vi "VITester_Global_Init.vi"(11 "Object":T1) -> ()   [LabVIEW 2013]
uses:
  <resource>/Framework/Providers/vitester-src/Support/VITester Project Item Ref.ctl
  <resource>/Framework/Providers/API/mxLvMenuItem.ctl
  <resource>/Framework/Providers/API/mxLvOverlayAlias.ctl
panel:
  out "error out":errorcluster
  in  "error in":errorcluster
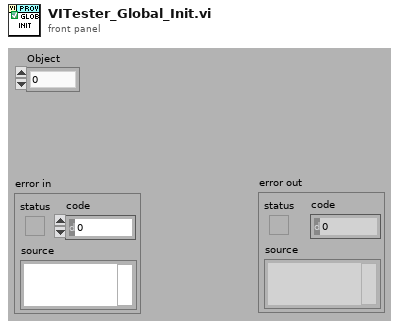
[diagram p1: front panel]
types:
  T1 = typedef "VITester Project Item Ref.ctl" = u64
  T2 = typedef "mxLvMenuItem.ctl" = cluster{"Menu Name":string, "Description":string, "Icon File Name":path, "Menu Tag":string, "Enabled":bool, "Checked":bool, "Separator":bool, "Batchable":bool, "Weight":i32, "Batch Mode (Ignored if Not Batchable)":enum32{"Show If All Items Support Command", "Show If Any Items Support Command"}, "Menu Location":enum32{"<None>", "Project", "Project / Build Specifications", "Tools", "Tools / Source Control", "Tools / Real-Time Module", "Help"}, "Exclude From Getting Started Window Menu":bool}
  T3 = typedef "ItemRef.ctl" = u64
  T4 = typedef "mxLvOverlayAlias.ctl" = cluster{"Overlay Alias":string, "Icon File Name":path}
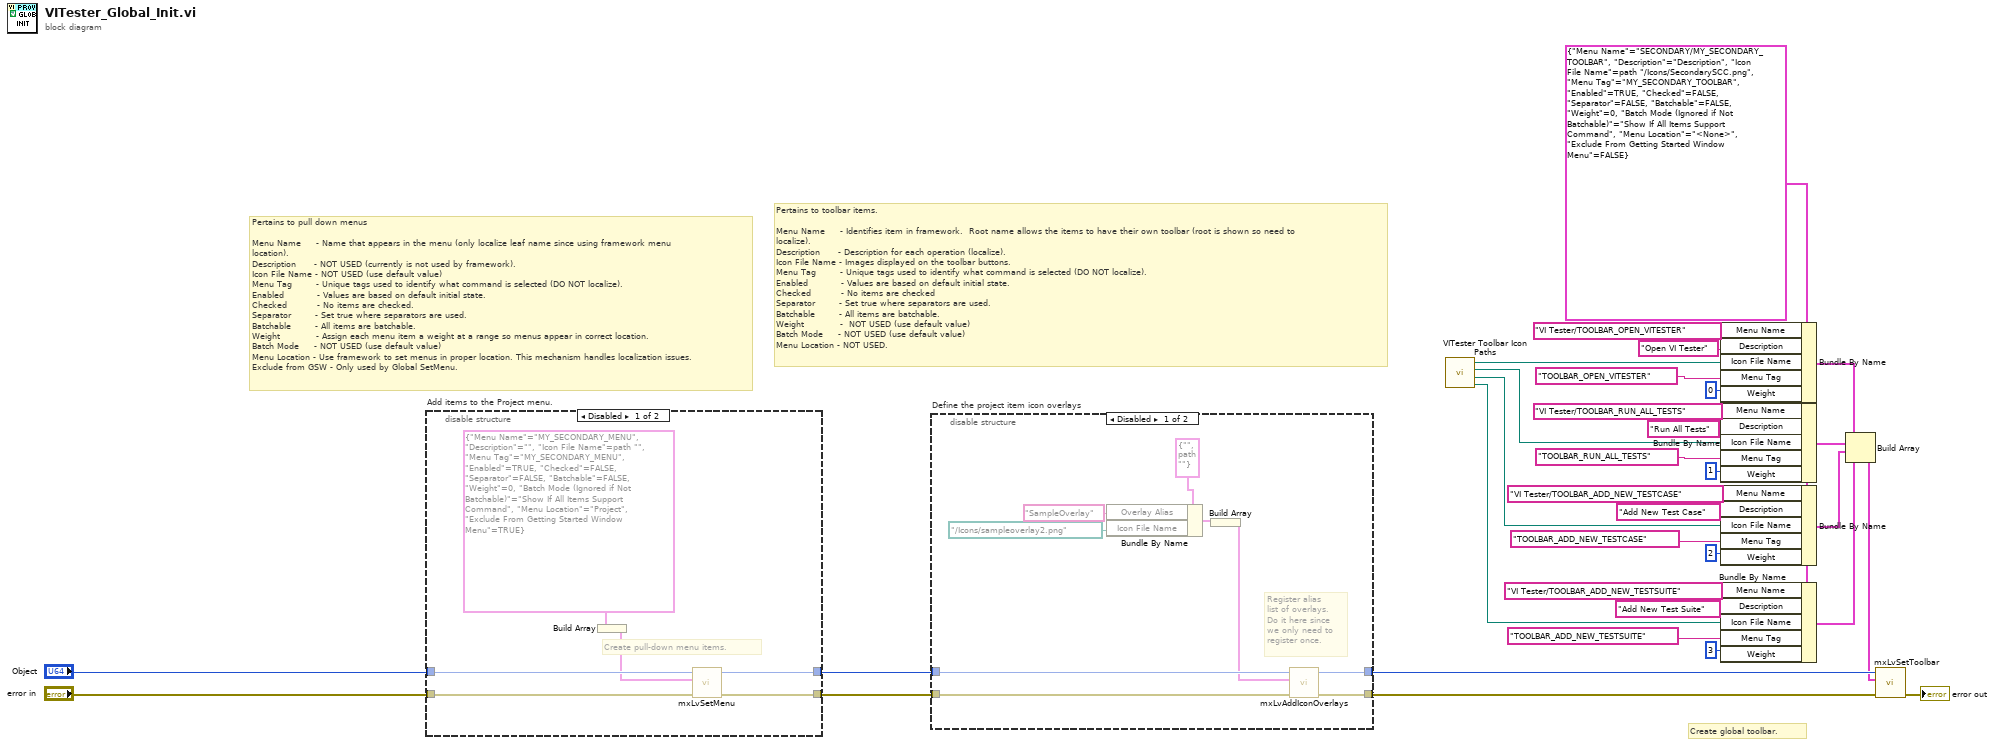
[diagram p0: block diagram]
diagram:
  w2 = T2 {"Menu Name"="SECONDARY/MY_SECONDARY_TOOLBAR", "Description"="Description", "Icon File Name"=path "../Icons/SecondarySCC.png", "Menu Tag"="MY_SECONDARY_TOOLBAR", "Enabled"=TRUE, "Checked"=FALSE, "Separator"=FALSE, "Batchable"=FALSE, "Weight"=0, "Batch Mode (Ignored if Not Batchable)"=enum."Show If All Items Support Command", "Menu Location"=enum."<None>", "Exclude From Getting Started Window Menu"=FALSE} ("Menu Item")
  # "Pertains to toolbar items.\n\nMenu Name     - Identifies item in framework.  Root name allows the items to have their own toolbar (root is shown so need to localize).\nDescription      - Description for each operation (localize).\nIcon File Name - Images displayed on the toolbar buttons.\nMenu Tag        - Unique tags used to identify what command is selected (DO NOT localize).\nEnabled           - Values are based on default initial state.\nChecked          - No items are checked\nSeparator        - Set true where separators are used.\nBatchable        - All items are batchable.\nWeight            -  NOT USED (use default value)\nBatch Mode     - NOT USED (use default value)\nMenu Location - NOT USED."
  # "Pertains to pull down menus\n\nMenu Name     - Name that appears in the menu (only localize leaf name since using framework menu location).\nDescription      - NOT USED (currently is not used by framework).\nIcon File Name - NOT USED (use default value)\nMenu Tag        - Unique tags used to identify what command is selected (DO NOT localize).\nEnabled           - Values are based on default initial state.\nChecked          - No items are checked.\nSeparator        - Set true where separators are used.\nBatchable        - All items are batchable.\nWeight            - Assign each menu item a weight at a range so menus appear in correct location.\nBatch Mode     - NOT USED (use default value)\nMenu Location - Use framework to set menus in proper location. This mechanism handles localization issues.\nExclude from GSW - Only used by Global SetMenu."
  # "Create global toolbar."
  n1 = disable-structure "Add items to the Project menu." shown="Disabled" {
    disable-tunnel: "error in" -> [w39 w40]
    disable-tunnel: [w38 w40] -> w32
    disable-tunnel: [w37 w41] -> w31
    disable-tunnel: "Object" -> [w36 w41]
    frame Disabled {
      # "Create pull-down menu items."
      n2 = Build Array(T2 {"Menu Name"="MY_SECONDARY_MENU", "Description"="", "Icon File Name"=path "", "Menu Tag"="MY_SECONDARY_MENU", "Enabled"=TRUE, "Checked"=FALSE, "Separator"=FALSE, "Batchable"=FALSE, "Weight"=0, "Batch Mode (Ignored if Not Batchable)"=enum."Show If All Items Support Command", "Menu Location"=enum."Project", "Exclude From Getting Started Window Menu"=TRUE} ("Menu Item")) -> (w34:T2[])
      n3 = call <resource>:"mxLvSetMenu.vi"("error in"=w39, "Menu Items"=w34, "Item"=w36) -> ("error out"=w38:errorcluster, "Item"=w37:T3)  [unwired: 7 in]
    }
    frame Enabled {
    }
  }
  n4 = disable-structure "Define the project item icon overlays" shown="Disabled" {
    disable-tunnel: w32 -> [w50 w51]
    disable-tunnel: w31 -> [w49 w52]
    disable-tunnel: [w48 w52] -> w30
    disable-tunnel: [w47 w51] -> w29
    frame Disabled {
      # "Register alias list of overlays.  Do it here since we only need to register once."
      n5 = Bundle By Name(cluster=T4 {"Overlay Alias"="", "Icon File Name"=path ""} ("Icon Overlay Alias"), "Overlay Alias"="SampleOverlay", "Icon File Name"=path "../Icons/sampleoverlay2.png") -> (w45:T4)
      n6 = Build Array(w45) -> (w44:T4[])
      n7 = call <resource>:"mxLvAddIconOverlays.vi"("error in"=w50, "Overlay Aliases"=w44, "Item"=w49) -> ("error out"=w47:errorcluster, "Item"=w48:T3)  [unwired: 7 in]
    }
    frame Enabled {
    }
  }
  n8 = call <resource>:"VITester Toolbar Icon Paths.vi"() -> ("Add New TestSuite toolbar icon"=w5:path, "Add New TestCase toolbar icon"=w17:path, "Run All Tests toolbar icon"=w12:path, "Open VI Tester toolbar icon"=w22:path)  [unwired: 8 in]
  n9 = Bundle By Name(cluster=w2, "Menu Name"="VI Tester/TOOLBAR_OPEN_VITESTER", "Description"="Open VI Tester", "Icon File Name"=w22, "Menu Tag"="TOOLBAR_OPEN_VITESTER", "Weight"=0) -> (w25:T2)
  n10 = Bundle By Name(cluster=w2, "Menu Name"="VI Tester/TOOLBAR_RUN_ALL_TESTS", "Description"="Run All Tests", "Icon File Name"=w12, "Menu Tag"="TOOLBAR_RUN_ALL_TESTS", "Weight"=1) -> (w1:T2)
  n11 = Bundle By Name(cluster=w2, "Menu Name"="VI Tester/TOOLBAR_ADD_NEW_TESTCASE", "Description"="Add New Test Case", "Icon File Name"=w17, "Menu Tag"="TOOLBAR_ADD_NEW_TESTCASE", "Weight"=2) -> (w9:T2)
  n12 = Bundle By Name(cluster=w2, "Menu Name"="VI Tester/TOOLBAR_ADD_NEW_TESTSUITE", "Description"="Add New Test Suite", "Icon File Name"=w5, "Menu Tag"="TOOLBAR_ADD_NEW_TESTSUITE", "Weight"=3) -> (w3:T2)
  n13 = Build Array(w25, w1, w9, w3) -> (w26:T2[])
  n14 = call <resource>:"mxLvSetToolbar.vi"("error in"=w29, "Toolbar Items"=w26, "Item"=w30) -> ("error out"=→"error out":errorcluster)  [unwired: 7 in, 1 out]
